vi "SetCurrent(General).vi"(8 "Error In":errorcluster, 10 "Current":dbl min=0.0 max=10.0 format="%.2g", 11 "VISA resource name":refnum<visa-resource-name>) -> (0 "Error Out":errorcluster, 3 "VISA resource name out":refnum<visa-resource-name>)   [LabVIEW 2013]
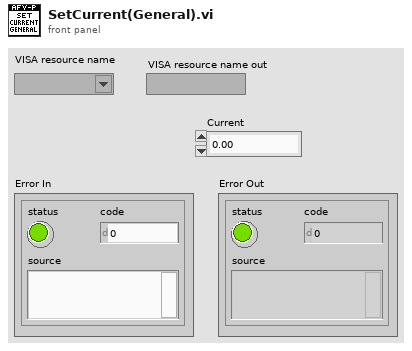
[diagram p1: front panel]
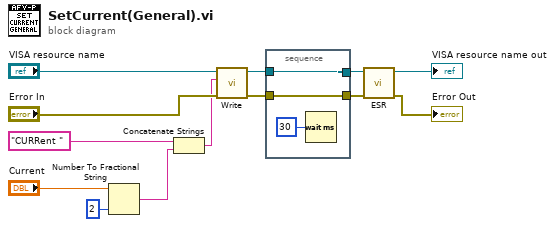
[diagram p0: block diagram]
diagram:
  n1 = Number To Fractional String(number="Current", precision (6)=i16 2) -> (F-format string=w7:string)  [unwired: 2 in]
  n2 = Concatenate Strings("CURRent " ("Write Buffer"), w7) -> (w8:string)
  n3 = call "Write.vi"("Error In"="Error In", "Write Buffer"=w8, "VISA resource name"="VISA resource name") -> ("Error Out"=w3:errorcluster, "VISA resource name out"=w4:refnum<visa-resource-name>)  [unwired: 7 in]
  n4 = stacked-sequence {
    tunnel: [w15] -> w6
    tunnel: w4 -> [w15]
    tunnel: [w14] -> w5
    tunnel: w3 -> [w14]
    frame #0 {
      n5 = Wait (ms)(milliseconds to wait=u32 30) -> ()  [unwired: 1 out]
    }
  }
  n6 = call "ESR.vi"("Error In"=w5, "VISA resource name"=w6) -> ("Error Out"=→"Error Out":errorcluster, "VISA resource name out"=→"VISA resource name out":refnum<visa-resource-name>)  [unwired: 8 in]
